vi "Unserialize.vi"(6 "All Build Configs":string[](array[string]), 8 "error in (no error)":errorcluster, 9 "Serialization Version":string, 10 "XML Node":refnum<class "XML Node.lvclass">, 11 "Caraya Item in":refnum<class "Caraya Item.lvclass">) -> (0 "error out":errorcluster, 2 "Invalid Version?":bool, 3 "Caraya Item out":refnum<class "Caraya Item.lvclass">)   [LabVIEW 2019, in "Caraya Library.lvlib" / "Caraya Item.lvclass"]
uses:
  Caraya Item.lvclass
  libs/Solution.lvlibp/Solution/XML Reader/XML Node.lvclass
  Caraya Item.lvclass/Caraya Item.ctl
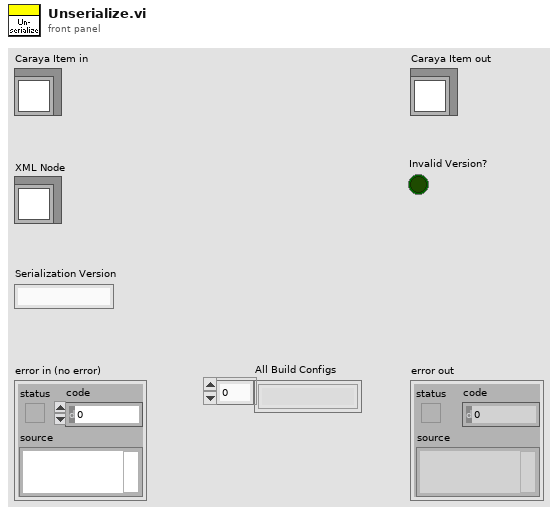
[diagram p1: front panel]
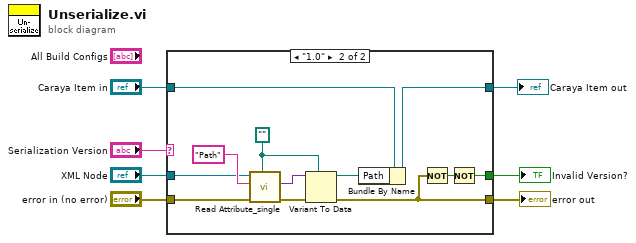
[diagram p0: block diagram]
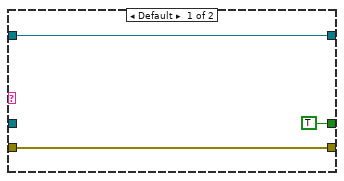
[diagram p2: hidden frame]
diagram:
  n1 = case shown="\"1.0\"" "Serialization Version" {
    tunnel: "XML Node" -> [_ w19]
    tunnel: "Caraya Item in" -> [w8 w16]
    tunnel: [w8 w15] -> w5
    tunnel: [TRUE w11] -> w4
    tunnel: [w9 w12] -> w3
    tunnel: "error in (no error)" -> [w9 w22]
    frame Default {
    }
    frame "1.0" {
      w17 = path ""
      n2 = call "Read Attribute_single.vi"("Type"=w17, "error in (no error)"=w22, "Name"="Path", "XML Reader in"=w19) -> ("error out"=w21:errorcluster, "Value"=w18:variant)  [unwired: 6 in]
      n3 = Variant To Data(error in=w21, type=w17, Variant=w18) -> (data=w14:path, error out=w12:errorcluster)
      n4 = Bundle By Name(cluster=w16, "Path"=w14) -> (w15:refnum<class "Caraya Item.lvclass">)
      n5 = Not(x=w12) -> (.not. x?=w13:bool)
      n6 = Not(x=w13) -> (.not. x?=w11:bool)
    }
  }
  "error out" <- w3
  "Invalid Version?" <- w4
  "Caraya Item out" <- w5
